vi "Windows Message Queue Size.vi"(0 "win msg queue":T1, 1 "error in (no error)":errorcluster) -> (2 "win msg queue out":T1, 3 "Items in queue":i32, 4 "error out":errorcluster)   [LabVIEW 2017, in "Windows messages for Labview (32 and 64).lvlib"]
doc: "Returns the number of messages waiting in the queue specified by win msg queue.\n\nErrors:\n6751: not a valid windows message queue."
uses:
  Windows messages for Labview (32 and 64).lvlib
  Win Msg Queue RefNum.ctl
  Windows Messages for LabVIEW_64.dll
  Windows Messages for LabVIEW_32.dll
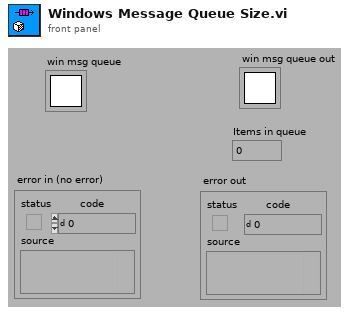
[diagram p1: front panel]
types:
  T1 = typedef "Windows messages for Labview (32 and 64).lvlib/Win Msg Queue RefNum.ctl" = refnum<k1>
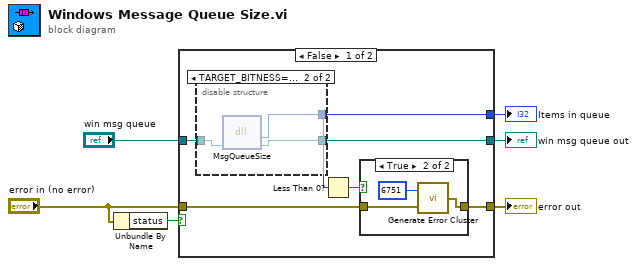
[diagram p0: block diagram]
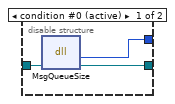
[diagram p2: hidden frame]
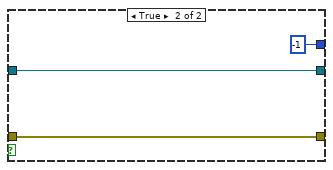
[diagram p4: hidden frame]
diagram:
  n1 = Unbundle By Name("error in (no error)") -> ("status"=w3:bool)
  n2 = case shown="False" w3 {
    tunnel: "win msg queue" -> [w9 w24]
    tunnel: [w7 -1] -> w1
    tunnel: "error in (no error)" -> [w11 w25]
    tunnel: [w10 w25] -> w4
    tunnel: [w8 w24] -> w2
    frame False {
      n3 = disable-structure shown="TARGET_BITNESS==32" {
        disable-tunnel: w9 -> [w15 w18]
        disable-tunnel: [w14 w17] -> w8
        disable-tunnel: [w13 w16] -> w7
        frame condition #0 (active) {
          n4 = dll-call lib="M:/_dev/progs/LabVIEW/_lib/Windows Messages for Labview/llb/Windows Messages for LabVIEW_64.dll" fn="MsgQueueSize"("occurrence"=w15) -> ("return type"=w13:i32, "occurrence"=w14:T1)  [unwired: 3 in, 2 out]
        }
        frame condition #1 {
          n5 = dll-call lib="D:/labview_d/temp/Windows Messaging/Windows Messages for Labview/llb/Windows Messages for LabVIEW_32.dll" fn="MsgQueueSize"("occurrence"=w18) -> ("return type"=w16:i32, "occurrence"=w17:T1)  [unwired: 3 in, 2 out]
        }
      }
      n6 = Less Than 0?(x=w7) -> (x < 0?=w12:bool)
      n7 = case shown="True" w12 {
        tunnel: [w19 w21] -> w10
        tunnel: w11 -> [w19 w22]
        frame False {
        }
        frame True {
          n8 = call "Generate Error Cluster.vi"("error in (no error)"=w22, "Error Code"=6751) -> ("error out"=w21:errorcluster)
        }
      }
    }
    frame True {
    }
  }
  "error out" <- w4
  "win msg queue out" <- w2
  "Items in queue" <- w1
